vi "Set DC Pins.vi"(8 "error in (no error)":errorcluster, 11 "Power Sweep In":refnum<class "Power Sweep.lvclass">) -> (0 "error out":errorcluster, 3 "Power Sweep Out":refnum<class "Power Sweep.lvclass">)   [LabVIEW 2018, in "Power Sweep.lvlib" / "Power Sweep.lvclass"]
uses:
  Power Sweep.lvclass
  C:/Sequence Automation/Plugins/Measurement Interface.lvlibp/Measurement Interface.lvclass
  Power Sweep.lvclass/Power Sweep.ctl
  Write PAE Pins.vi
  Plugins/Measurement Interface.lvlibp/Private Methods/Measurement Parameters/Read Measurement Parameters.vi
  Write DC Pins.vi
  Plugins/String Database.lvlibp/String Database.lvclass
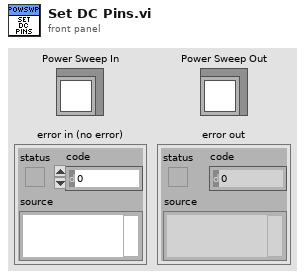
[diagram p1: front panel]
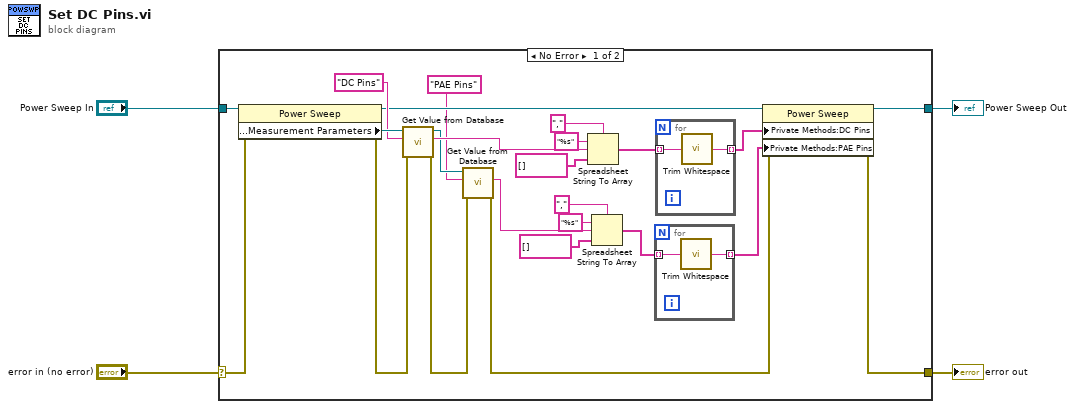
[diagram p0: block diagram]
diagram:
  n1 = case shown="No Error" "error in (no error)" {
    selector: "error in (no error)" -> [w28 w34]
    tunnel: [w18 w34] -> w3
    tunnel: [w16 w33] -> w1
    tunnel: "Power Sweep In" -> [w27 w33]
    frame No Error {
      n2 = property class="Power Sweep"(reference=w27, error in=w28) -> (reference out=w17:refnum<class "Power Sweep.lvclass">, error out=w25:errorcluster, "Protected Methods:Measurement Parameters"=w26:refnum<class "String Database.lvclass">)
      n3 = call "Get Value from Database.vi"("error in (no error)"=w25, "Entry Name"="DC Pins", "Message in"=w26) -> ("error out"=w12:errorcluster, "Entry Value"=w21:string, "Message out"=w14:refnum<class "String Database.lvclass">)  [unwired: 5 in, 1 out]
      n4 = call "Get Value from Database.vi"("error in (no error)"=w12, "Entry Name"="PAE Pins", "Message in"=w14) -> ("error out"=w11:errorcluster, "Entry Value"=w6:string)  [unwired: 5 in, 2 out]
      n5 = Spreadsheet String To Array(delimiter (Tab)=",", format string="%s", spreadsheet string=w21, array type (2D Dbl)=string[] []) -> (array=w19:string[])
      n6 = Spreadsheet String To Array(delimiter (Tab)=",", format string="%s", spreadsheet string=w6, array type (2D Dbl)=string[] []) -> (array=w10:string[])
      n7 = for {
        tunnel: w10 -> [w30] mode=indexing
        tunnel: [w29] -> w5 mode=indexing
        n8 = call <vilib>:"Trim Whitespace.vi"("string"=w30) -> ("trimmed string"=w29:string)  [unwired: 1 in]
      }
      n9 = for {
        tunnel: w19 -> [w32] mode=indexing
        tunnel: [w31] -> w15 mode=indexing
        n10 = call <vilib>:"Trim Whitespace.vi"("string"=w32) -> ("trimmed string"=w31:string)  [unwired: 1 in]
      }
      n11 = property class="Power Sweep"(reference=w17, error in=w11, "Private Methods:DC Pins"=w15, "Private Methods:PAE Pins"=w5) -> (reference out=w16:refnum<class "Power Sweep.lvclass">, error out=w18:errorcluster)
    }
    frame Error {
    }
  }
  "error out" <- w3
  "Power Sweep Out" <- w1
